vi "Test - Using Traverse.vi"   [LabVIEW 2020]
doc: "本测试VI由Using Traverse.vi范例使用。"
uses:
  <vilib>/Utility/file.llb/Write Delimited Spreadsheet (DBL).vi
panel:
  # "请不要保存对本VI的改动！！！本VI为Using Traverse.vi范例VI的操作目标VI。因此，保存本VI的改动可能会使Using Traverse.vi范例无法演示其预定的功能。"
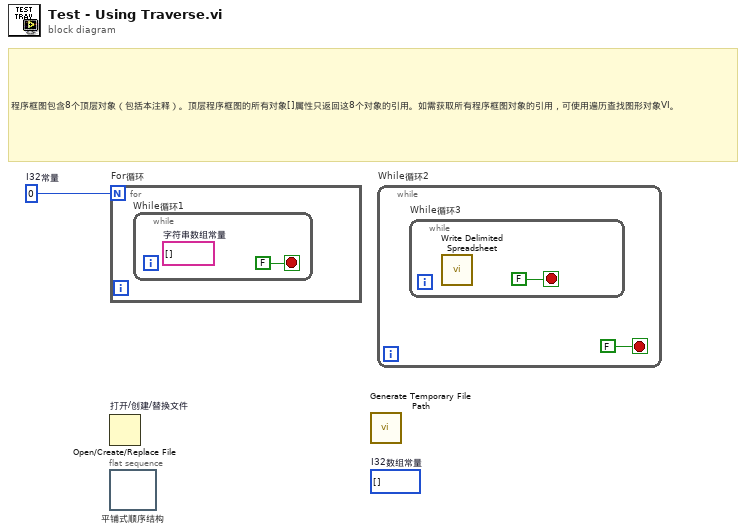
[diagram p0: block diagram]
diagram:
  w1 = 0  # I32常量
  (unwired) i32[] []  # I32数组常量
  # "程序框图包含8个顶层对象（包括本注释）。顶层程序框图的所有对象[]属性只返回这8个对象的引用。如需获取所有程序框图对象的引用，可使用遍历查找图形对象VI。"
  n1 = Open/Create/Replace File "打开/创建/替换文件"() -> ()  [unwired: 6 in, 3 out]
  n2 = flat-sequence "平铺式顺序结构" {
    frame #0 {
    }
  }
  n3 = for "For循环" {
    N: w1 -> [_]
    n4 = while "While循环1" {
      stop <- FALSE stop-if-true
      (unwired) string[] []  # 字符串数组常量
    }
  }
  n5 = call <vilib>:"Generate Temporary File Path.vi"() -> ()  [unwired: 10 in, 2 out]
  n6 = while "While循环2" {
    stop <- FALSE stop-if-true
    n7 = while "While循环3" {
      stop <- FALSE stop-if-true
      n8 = call-poly <vilib>:"Write Delimited Spreadsheet.vi"() -> ()  [unwired: 14 in, 2 out]
    }
  }
